vi "Wait for Message (blocking).vi"(8 "error in (no error)":errorcluster, 9 "timeout in ms (-1)":i32=-1, 10 "Command":string, 11 "Listening queue in":refnum<queue>) -> (0 "error out":errorcluster, 1 "Message Data":variant, 2 "Message":string, 3 "Listening queue out":refnum<queue>)   [LabVIEW 2020, in "Generic Plugin.lvclass"]
doc: "Waits for a message with the specified command, ignoring all other messages. This is a blocking VI. This VI can be given a timeout value (-1 for no timeout) so it only blocks for a set amount of time. If no message is received, the message \"Timeout\" with no data will be returned."
uses:
  Generic Plugin.lvclass
  Generic Plugin.lvclass/Generic Plugin.ctl
  Sub VIs/Message Queue/test Message Queue.lvlib
  Sub VIs/Message Queue/Message Cluster.ctl
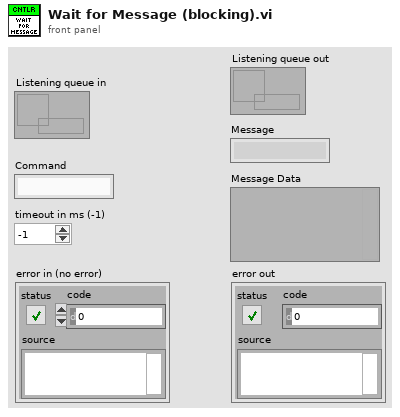
[diagram p1: front panel]
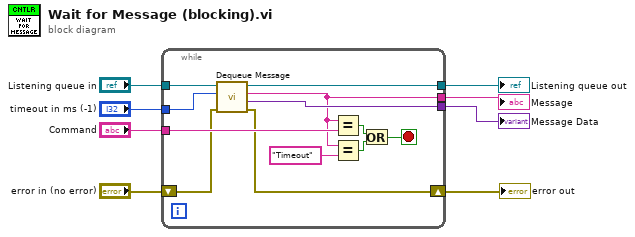
[diagram p0: block diagram]
diagram:
  n1 = while {
    tunnel: "Listening queue in" -> [w20]
    tunnel: "Command" -> [w19]
    tunnel: [w18] -> w4
    shift-right: [w16] -> w8
    shift-left: "error in (no error)" -> [w17]
    tunnel: [w13] -> w3
    tunnel: [w15] -> w2
    tunnel: "timeout in ms (-1)" -> [w14]
    stop <- w9 stop-if-true
    n2 = call "Dequeue Message.vi"("error in (no error)"=w17, "timeout in ms (-1)"=w14, "Message Queue"=w20) -> ("error out"=w16:errorcluster, "Message Data"=w15:variant, "Message"=w13:string, "dup Message Queue"=w18:refnum<queue>)  [unwired: 5 in]
    n3 = Equal?(x=w13, y=w19) -> (x = y?=w11:bool)
    n4 = Equal?(x=w13, y="Timeout") -> (x = y?=w10:bool)
    n5 = Or(x=w11, y=w10) -> (x .or. y?=w9:bool)
  }
  "error out" <- w8
  "Listening queue out" <- w4
  "Message" <- w3
  "Message Data" <- w2
